vi "Labview_USB_ADC_Test.vi"() -> ()   [LabVIEW 2012]
uses:
  Ginkgo GPIO/Labview_USB_GPIO_Test/lib/labview_32bit/ControlI2C/Ginkgo_Driver.dll
panel:
  in  "stop":bool
  out "error out":errorcluster
  out "CH7":dbl(knob) scale=0.0..3.3
  out "CH6":dbl(knob) scale=0.0..3.3
  out "CH5":dbl(knob) scale=0.0..3.3
  out "CH4":dbl(knob) scale=0.0..3.3
  out "CH3":dbl(knob) scale=0.0..3.3
  out "CH2":dbl(knob) scale=0.0..3.3
  out "CH1":dbl(knob) scale=0.0..3.3
  out "CH0":dbl(knob) scale=0.0..3.3
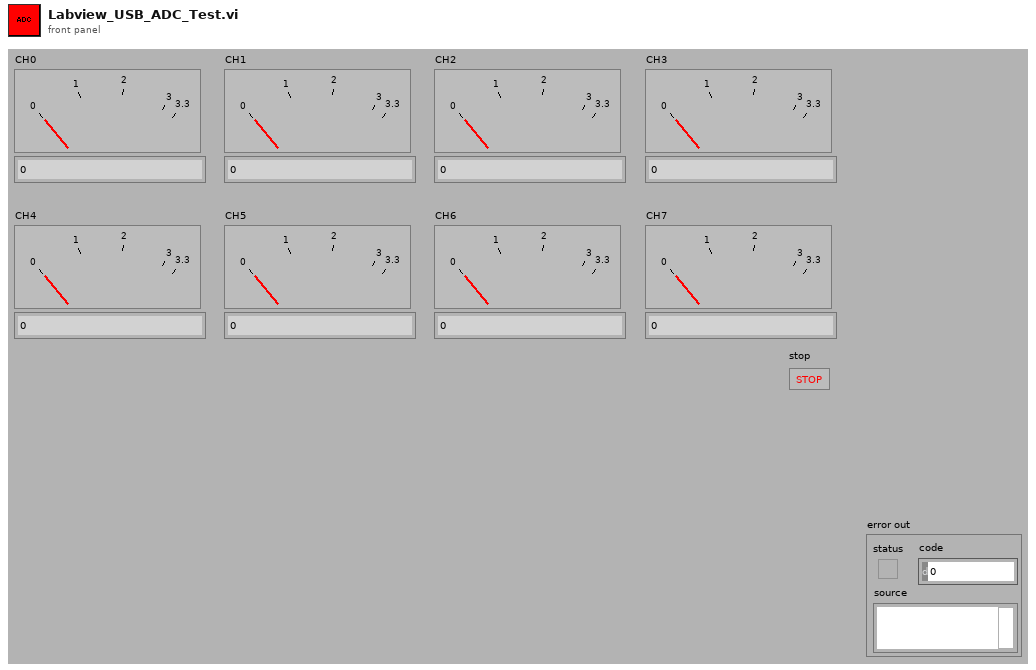
[diagram p1: front panel]
types:
  T1 = enum16{"Init", "ScanDevice", "OpenDevice", "InitDevice", "Read data", "Idel", "Error"}
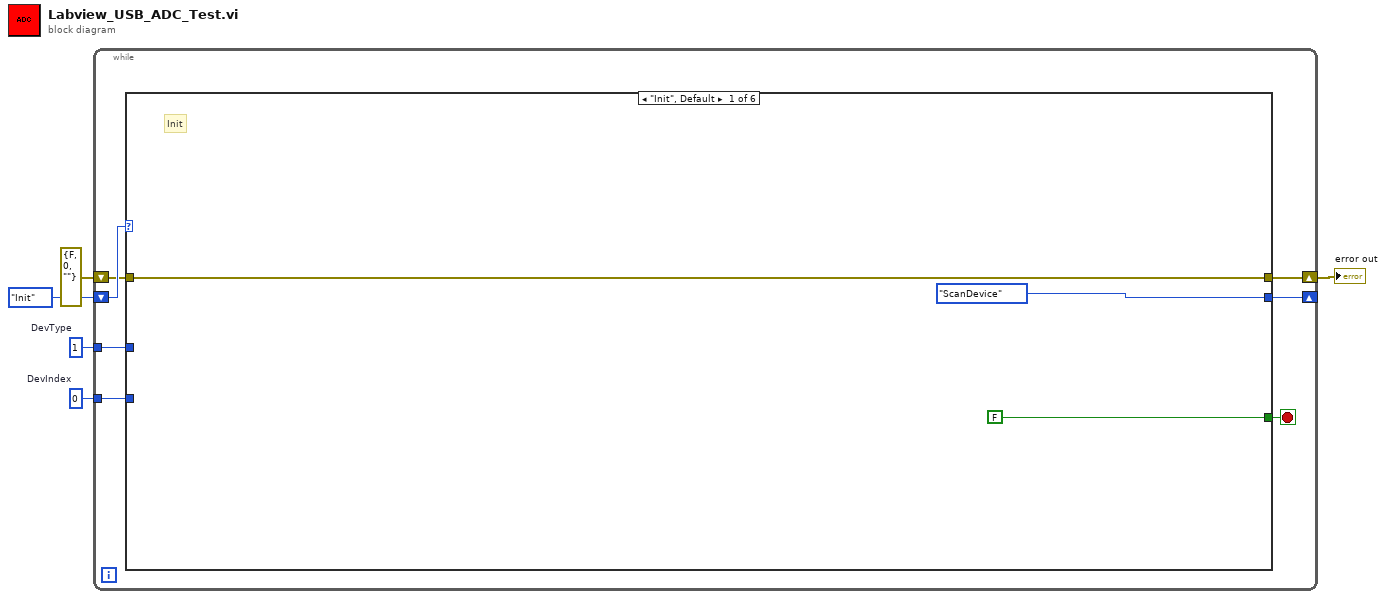
[diagram p0: block diagram]
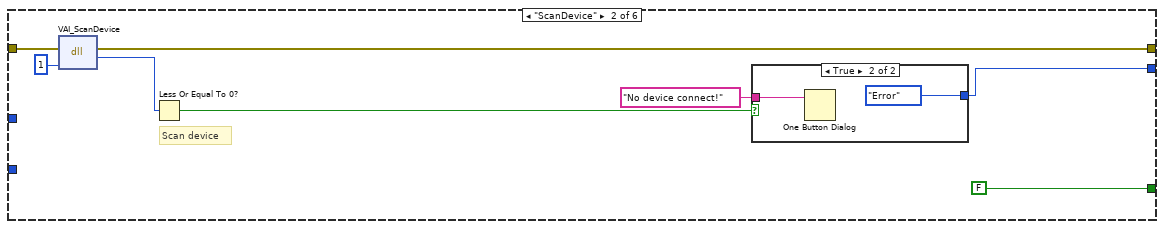
[diagram p2: hidden frame]
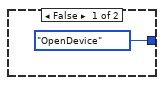
[diagram p3: hidden frame]
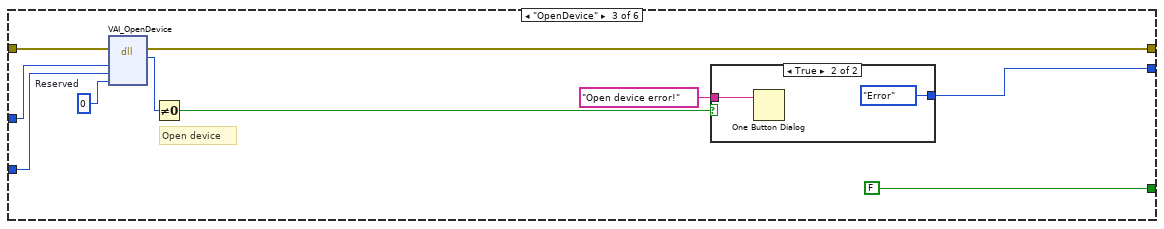
[diagram p4: hidden frame]
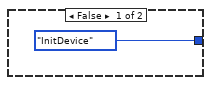
[diagram p5: hidden frame]
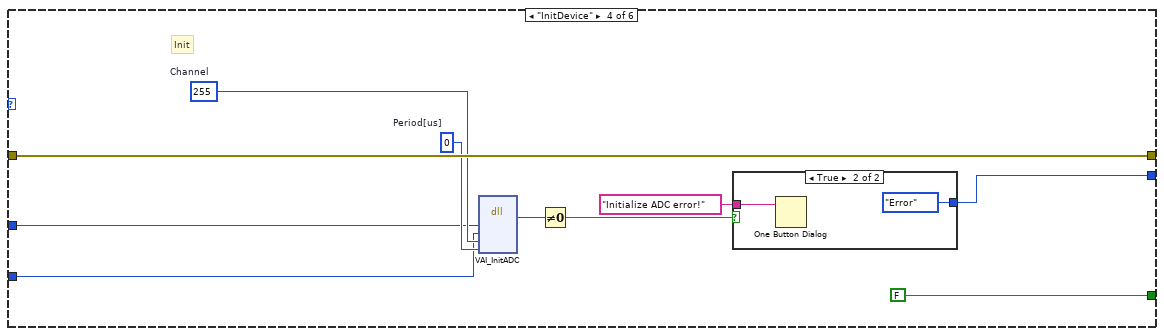
[diagram p6: hidden frame]
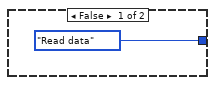
[diagram p7: hidden frame]
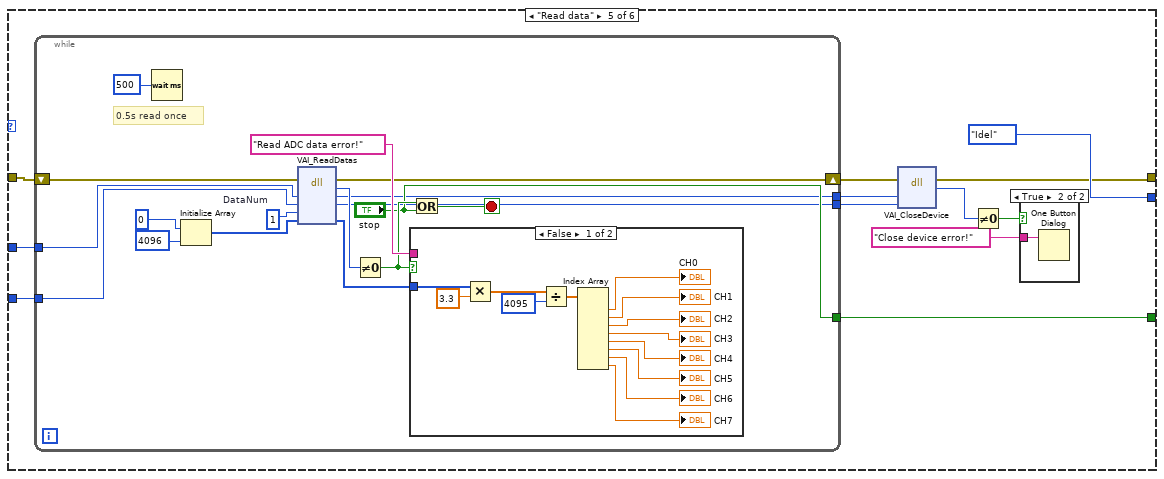
[diagram p8: hidden frame]
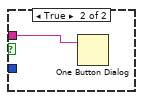
[diagram p10: hidden frame]
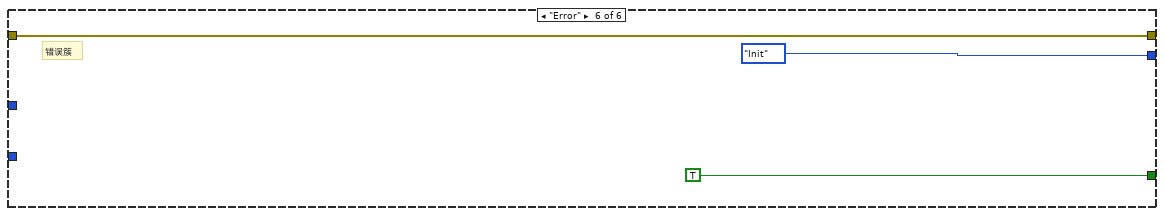
[diagram p11: hidden frame]
diagram:
  w1 = 0  # DevIndex
  w2 = 1  # DevType
  n1 = while {
    shift-right: [w12] -> _
    shift-left: T1."Init" ("Enum") -> [w11]
    shift-right: [w9] -> w3
    shift-left: errorcluster {"status"=FALSE, "code"=0, "source"=""} ("error out") -> [w8]
    tunnel: w2 -> [w7]
    tunnel: w1 -> [w6]
    stop <- w10 stop-if-true
    n2 = case shown="\"Init\", Default" w11 {
      tunnel: [T1."ScanDevice" ("Enum") w19 w33 w46 T1."Idel" ("Enum") T1."Init" ("Enum")] -> w12
      tunnel: [FALSE ("stop") FALSE ("stop") FALSE ("stop") FALSE ("stop") w63 TRUE ("stop")] -> w10
      tunnel: [w13 w17 w30 w44 w57 w97] -> w9
      tunnel: w8 -> [w13 w16 w31 w44 w62 w97]
      tunnel: w7 -> [_ _ w28 w41 w56 _]
      tunnel: w6 -> [_ _ w27 w40 w55 _]
      frame "Init", Default {
        # "Init"
      }
      frame "ScanDevice" {
        # "Scan device"
        n3 = dll-call lib="E:/Project/vt_ginkgo/truck/Ginkgo Application Example/Labview/Ginkgo GPIO/Labview_USB_GPIO_Test/lib/labview_32bit/ControlI2C/Ginkgo_Driver.dll" fn="VAI_ScanDevice"(error in=w16, "NeedInit"=u8 1) -> (error out=w17:errorcluster, "return type"=w22:i32)  [unwired: 3 in, 1 out]
        n4 = Less Or Equal To 0?(x=w22) -> (x <= 0?=w21:bool)
        n5 = case shown="True" w21 {
          tunnel: "No device connect!" ("message") -> [_ w26]
          tunnel: [T1."OpenDevice" ("Enum") T1."Error" ("Enum")] -> w19
          frame False {
          }
          frame True {
            n6 = One Button Dialog(message=w26) -> ()  [unwired: 1 in, 1 out]
          }
        }
      }
      frame "OpenDevice" {
        w29 = 0  # Reserved
        # "Open device"
        n7 = dll-call lib="E:/Project/vt_ginkgo/truck/Ginkgo Application Example/Labview/Ginkgo GPIO/Labview_USB_GPIO_Test/lib/labview_32bit/ControlI2C/Ginkgo_Driver.*" fn="VAI_OpenDevice"(error in=w31, "DevType"=w28, "DevIndex"=w27, "Reserved"=w29) -> (error out=w30:errorcluster, "return type"=w35:i32)  [unwired: 5 in, 1 out]
        n8 = Not Equal To 0?(x=w35) -> (x != 0?=w34:bool)
        n9 = case shown="True" w34 {
          tunnel: "Open device error!" ("message") -> [_ w39]
          tunnel: [T1."InitDevice" ("Enum") T1."Error" ("Enum")] -> w33
          frame False {
          }
          frame True {
            n10 = One Button Dialog(message=w39) -> ()  [unwired: 1 in, 1 out]
          }
        }
      }
      frame "InitDevice" {
        w42 = u16 0  # Period[us]
        w43 = u8 255  # Channel
        # "Init"
        n11 = dll-call lib="E:/Project/vt_ginkgo/truck/Ginkgo Application Example/Labview/Ginkgo GPIO/Labview_USB_GPIO_Test/lib/labview_32bit/ControlI2C/Ginkgo_Driver.*" fn="VAI_InitADC"("DevType"=w41, "DevIndex"=w40, "Channel"=w43, "Period"=w42) -> ("return type"=w48:i32)  [unwired: 7 in, 2 out]
        n12 = Not Equal To 0?(x=w48) -> (x != 0?=w47:bool)
        n13 = case shown="True" w47 {
          tunnel: "Initialize ADC error!" ("message") -> [_ w52]
          tunnel: [T1."Read data" ("Enum") T1."Error" ("Enum")] -> w46
          frame False {
          }
          frame True {
            n14 = One Button Dialog(message=w52) -> ()  [unwired: 1 in, 1 out]
          }
        }
      }
      frame "Read data" {
        n15 = while {
          tunnel: ["stop"] -> w63
          shift-right: [w71] -> w61
          shift-left: w62 -> [w72]
          tunnel: w56 -> [w69]
          tunnel: w55 -> [w68]
          tunnel: [w67] -> w54
          tunnel: [w66] -> w53
          stop <- w74 stop-if-true
          w82 = u16 1  # DataNum
          # "0.5s read once"
          n16 = Wait (ms)(milliseconds to wait=u32 500) -> ()  [unwired: 1 out]
          n17 = Initialize Array(u16 0, 4096 ("dimension size")) -> (w80:u16[])
          n18 = dll-call lib="E:/Project/vt_ginkgo/truck/Ginkgo Application Example/Labview/Ginkgo GPIO/Labview_USB_GPIO_Test/lib/labview_32bit/ControlI2C/Ginkgo_Driver.dll" fn="VAI_ReadDatas"(error in=w72, "DevType"=w69, "DevIndex"=w68, "DataNum"=w82, "pData"=w80) -> (error out=w71:errorcluster, "return type"=w79:i32, "DevType"=w67:i32, "DevIndex"=w66:i32, "pData"=w76:u16[])  [unwired: 3 in, 1 out]
          n19 = Not Equal To 0?(x=w79) -> (x != 0?=w75:bool)
          n20 = case shown="False" w75 {
            tunnel: "Read ADC data error!" ("message") -> [_ w96]
            tunnel: w76 -> [w95 _]
            frame False {
              n21 = Multiply(x=w95, y=3.3) -> (x*y=w93:dbl[])
              n22 = Divide(x=w93, y=4095) -> (x/y=w91:dbl[])
              n23 = Index Array(array=w91) -> (element #1=→"CH0":dbl, element #2=→"CH1":dbl, element #3=→"CH2":dbl, element #4=→"CH3":dbl, element #5=→"CH4":dbl, element #6=→"CH5":dbl, element #7=→"CH6":dbl, element #8=→"CH7":dbl)  [unwired: 8 in]
            }
            frame True {
              n24 = One Button Dialog(message=w96) -> ()  [unwired: 1 in, 1 out]
            }
          }
          n25 = Or(x=w75, y="stop") -> (x .or. y?=w74:bool)
        }
        n26 = dll-call lib="E:/Project/vt_ginkgo/truck/Ginkgo Application Example/Labview/Ginkgo GPIO/Labview_USB_GPIO_Test/lib/labview_32bit/ControlI2C/Ginkgo_Driver.dll" fn="VAI_CloseDevice"(error in=w61, "DevType"=w54, "DevIndex"=w53) -> (error out=w57:errorcluster, "return type"=w60:i32)  [unwired: 4 in, 1 out]
        n27 = Not Equal To 0?(x=w60) -> (x != 0?=w59:bool)
        n28 = case shown="True" w59 {
          tunnel: "Close device error!" ("message") -> [_ w65]
          frame False {
          }
          frame True {
            n29 = One Button Dialog(message=w65) -> ()  [unwired: 1 in, 1 out]
          }
        }
      }
      frame "Error" {
        # "错误簇"
      }
    }
  }
  "error out" <- w3
